vi "get_resolution.vi"(8 "error in (no error)":errorcluster, 11 "ScanModeMG090624Camera in":refnum<class "ImagingModeMG090624Camera.lvclass">) -> (0 "error out":errorcluster, 1 "y":i32, 2 "x":i32, 3 "ScanModeMG090624Camera out":refnum<class "ImagingModeMG090624Camera.lvclass">)   [LabVIEW 2010, in "ImagingModeMG090624Camera.lvclass"]
uses:
  ImagingModeMG090624Camera.lvclass
  ImagingModeMG090624Camera.lvclass/ImagingModeMG090624Camera.ctl
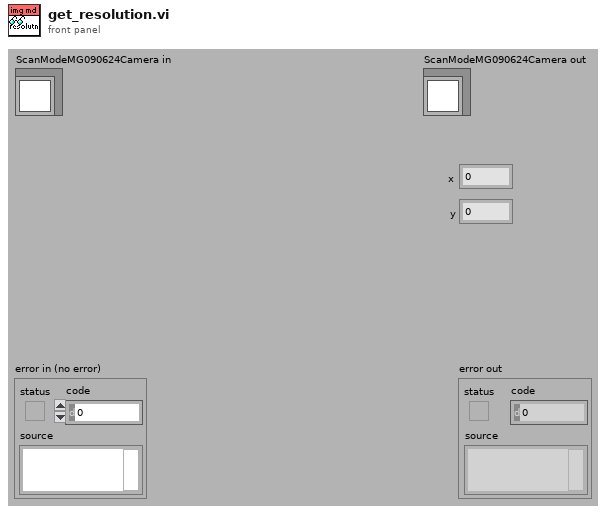
[diagram p1: front panel]
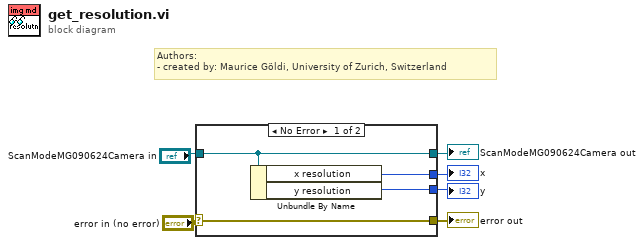
[diagram p0: block diagram]
diagram:
  # "Authors: \n- created by: Maurice Göldi, University of Zurich, Switzerland"
  n1 = case shown="No Error" "error in (no error)" {
    selector: "error in (no error)" -> [w10 w12]
    tunnel: [w10 w12] -> w5
    tunnel: [w9 w11] -> w2
    tunnel: "ScanModeMG090624Camera in" -> [w9 w11]
    tunnel: [w8 _] -> w4
    tunnel: [w7 _] -> w3
    frame No Error {
      n2 = Unbundle By Name(w9) -> ("x resolution"=w8:i32, "y resolution"=w7:i32)
    }
    frame Error {
    }
  }
  "error out" <- w5
  "x" <- w4
  "y" <- w3
  "ScanModeMG090624Camera out" <- w2
